vi "表格自动滚动显示.vi"(9 "显示行数":u32, 11 "表格控件":refnum<vi>) -> ()   [LabVIEW 2017]
uses:
  <vilib>/Utility/miscctls.llb/LVRowAndColumnUnsignedTypeDef.ctl
panel:
  in  "表格1":string[][](table)
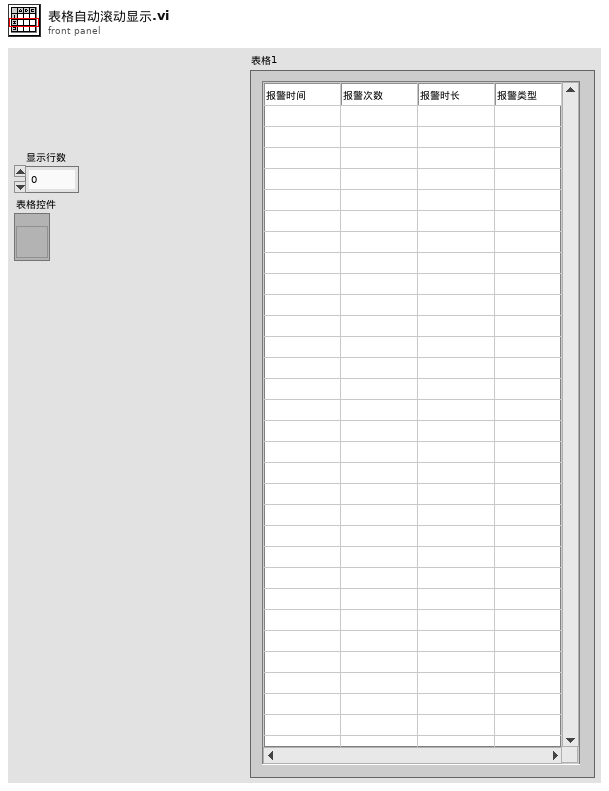
[diagram p1: front panel]
types:
  T1 = typedef "LVRowAndColumnUnsignedTypeDef.ctl" = cluster{"Row":u32, "Column":u32}
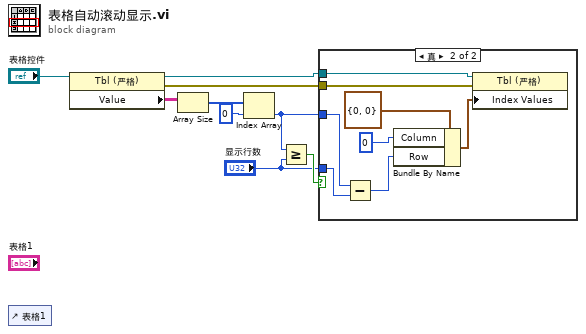
[diagram p0: block diagram]
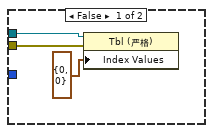
[diagram p2: hidden frame]
diagram:
  n1 = control-ref of="表格1"() -> ()  [unwired: 1 out]
  n2 = property class="Tbl (严格)"(reference="表格控件") -> (reference out=w5:refnum<vi>, error out=w1:errorcluster, "Value"=w9:string[][])  [unwired: 1 in]
  n3 = Array Size(array=w9) -> (size(s)=w8:i32[])
  n4 = Index Array(array=w8, index=0 ("索引")) -> (element=w3:i32)
  n5 = Greater Or Equal?(x=w3, y="显示行数") -> (x >= y?=w6:bool)
  n6 = case shown="真" w6 {
    tunnel: w5 -> [w12 w20]
    tunnel: "显示行数" -> [_ w15]
    tunnel: w3 -> [_ w16]
    tunnel: w1 -> [w10 w13]
    frame False {
      n7 = property class="Tbl (严格)"(reference=w12, error in=w10, "Index Values"=T1 {"Row"=0, "Column"=0} ("索引值")) -> ()  [unwired: 2 out]
    }
    frame True {
      n8 = Subtract(x=w16, y=w15) -> (x-y=w14:u32)
      n9 = Bundle By Name(cluster=T1 {"Row"=0, "Column"=0} ("索引值"), "Column"=u32 0, "Row"=w14) -> (w18:T1)
      n10 = property class="Tbl (严格)"(reference=w20, error in=w13, "Index Values"=w18) -> ()  [unwired: 2 out]
    }
  }
